vi "MixAndDownsample_5160.vi"(9 "Sine in":fxp<+/-,16,0>, 10 "Cosine in":fxp<+/-,16,0>, 11 "Sample in":i16) -> (0 "valid out":bool, 2 "Q out":fxp<+/-,16,14>, 3 "I out":fxp<+/-,16,14>)   [LabVIEW 2013]
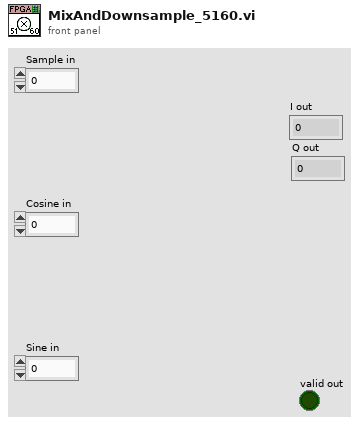
[diagram p1: front panel]
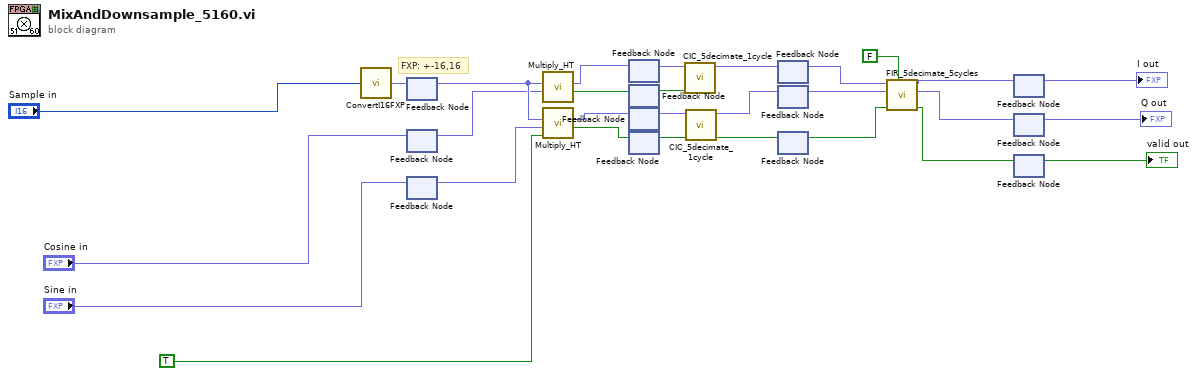
[diagram p0: block diagram]
diagram:
  # "FXP: +-16,16"
  n1 = call "ConvertI16FXP.vi"("I16"="Sample in") -> ("y"=w25:fxp<+/-,16,16>)
  n2 = feedback #1() -> (w26:fxp<+/-,16,16>)  [unwired: 1 in]
  n3 = feedback-in #1(w25) -> ()
  n4 = feedback #2() -> (w22:fxp<+/-,16,0>)  [unwired: 1 in]
  n5 = feedback-in #2("Cosine in") -> ()
  n6 = feedback #3() -> (w20:fxp<+/-,16,0>)  [unwired: 1 in]
  n7 = feedback-in #3("Sine in") -> ()
  n8 = call "Multiply_HT.vi"("DDS sample"=w22, "Signal sample"=w26) -> ("output valid"=w15:bool, "Output"=w13:fxp<+/-,16,14>)  [unwired: 8 in]
  n9 = call "Multiply_HT.vi"("Input Valid (T)"=TRUE ("valid in"), "DDS sample"=w20, "Signal sample"=w26) -> ("output valid"=w18:bool, "Output"=w5:fxp<+/-,16,14>)  [unwired: 7 in]
  n10 = feedback #4() -> (w12:fxp<+/-,16,14>)  [unwired: 1 in]
  n11 = feedback-in #4(w13) -> ()
  n12 = feedback #5() -> (w14:bool)  [unwired: 1 in]
  n13 = feedback-in #5(w15) -> ()
  n14 = feedback #6() -> (w17:fxp<+/-,16,14>)  [unwired: 1 in]
  n15 = feedback-in #6(w5) -> ()
  n16 = feedback #7() -> (w16:bool)  [unwired: 1 in]
  n17 = feedback-in #7(w18) -> ()
  n18 = call "CIC_5decimate_1cycle.vi"("valid in"=w14, "Data in"=w12) -> ("Data out"=w11:fxp<+/-,16,14>)  [unwired: 7 in, 2 out]
  n19 = call "CIC_5decimate_1cycle.vi"("valid in"=w16, "Data in"=w17) -> ("valid out"=w7:bool, "Data out"=w8:fxp<+/-,16,14>)  [unwired: 7 in, 1 out]
  n20 = feedback #8() -> (w10:fxp<+/-,16,14>)  [unwired: 1 in]
  n21 = feedback-in #8(w11) -> ()
  n22 = feedback #9() -> (w9:fxp<+/-,16,14>)  [unwired: 1 in]
  n23 = feedback-in #9(w8) -> ()
  n24 = feedback #10() -> (w6:bool)  [unwired: 1 in]
  n25 = feedback-in #10(w7) -> ()
  n26 = call "FIR_5decimate_5cycles.vi"("reset"=FALSE, "valid in"=w6, "Q in"=w9, "I in"=w10) -> ("valid out"=w2:bool, "Q out"=w3:fxp<+/-,16,14>, "I out"=w4:fxp<+/-,16,14>)  [unwired: 4 in, 1 out]
  n27 = feedback #11() -> (→"I out":fxp<+/-,16,14>)  [unwired: 1 in]
  n28 = feedback-in #11(w4) -> ()
  n29 = feedback #12() -> (→"Q out":fxp<+/-,16,14>)  [unwired: 1 in]
  n30 = feedback-in #12(w3) -> ()
  n31 = feedback #13() -> (→"valid out":bool)  [unwired: 1 in]
  n32 = feedback-in #13(w2) -> ()
